vi "Read Attributes.vi"(11 "Sequence Msg":refnum<class "Sequence Msg.lvclass">) -> (2 "Payload":T1)   [LabVIEW 2019, in "Sequence.lvlib" / "Sequence Msg.lvclass"]
uses:
  Sequence Msg.lvclass
  Sequence Msg.lvclass/Sequence Msg.ctl
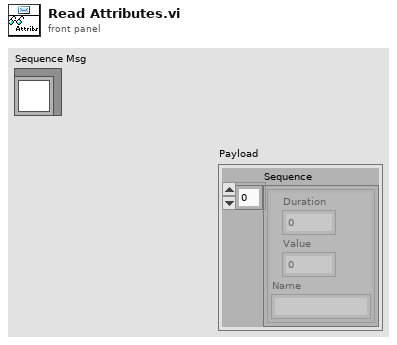
[diagram p1: front panel]
types:
  T1 = cluster{"Sequence":cluster{"Duration":i32, "Value":u32, "Name":string}[]}
  T2 = cluster{"Duration":i32, "Value":u32, "Name":string}[]
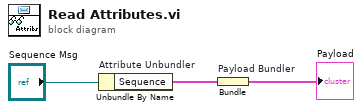
[diagram p0: block diagram]
diagram:
  n1 = Unbundle By Name "Attribute Unbundler"("Sequence Msg") -> ("Sequence"=w1:T2)
  n2 = Bundle "Payload Bundler"("Sequence"=w1) -> (→"Payload":T1)  [unwired: 1 in]
